vi "NML Async Lock.vi"(8 "error in (no error)":errorcluster, 11 "VISA Refnum in":refnum<visa-resource-name>) -> (0 "error out":errorcluster, 2 "Timeout":u32, 3 "VISA Refnum out":refnum<visa-resource-name>)   [LabVIEW 2025]
doc: "Gets Timeout value and Async Resource Lock. However, if connection fails it reopens connection and retrys.\nAuthor: Scott Hannahs <sth@magnet.fsu.edu>\n\nThis software is licensed for use under the “MIT License\"\nCopyright (c) 2025 Scott Hannahs, sth@sth@magnet.sthnet.net\n\nPermission is hereby granted, free of charge, to any person obtaining a copy of this software and associated documentation files (the \"Software\"), to deal in the Software without restriction, including without limitation the rights to use, copy, modify, merge, publish, distribute, sublicense, and/or sell copies of the Software, and to permit persons to whom the Software is furnished to do so, subject to the following conditions: The above copyright notice and this permission notice shall be included in all copies or substantial portions of the Software.\n\nTHE SOFTWARE IS PROVIDED \"AS IS\", WITHOUT WARRANTY OF ANY KIND, EXPRESS OR IMPLIED, INCLUDING BUT NOT LIMITED TO THE WARRANTIES OF MERCHANTABILITY, FITNESS FOR A PARTICULAR PURPOSE AND NONINFRINGEMENT. IN NO EVENT SHALL THE AUTHORS OR COPYRIGHT HOLDERS BE LIABLE FOR ANY CLAIM, DAMAGES OR OTHER LIABILITY, WHETHER IN AN ACTION OF CONTRACT, TORT OR OTHERWISE, ARISING FROM, OUT OF OR IN CONNECTION WITH THE SOFTWARE OR THE USE OR OTHER DEALINGS IN THE SOFTWARE."
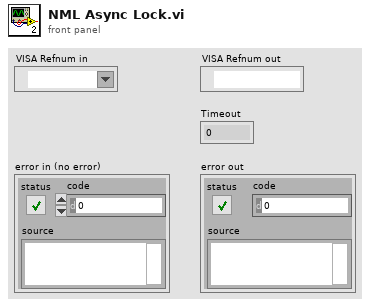
[diagram p1: front panel]
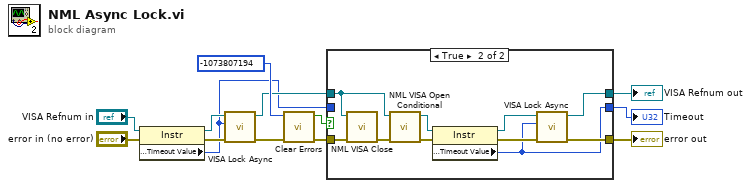
[diagram p0: block diagram]
diagram:
  n1 = property class="Instr"(reference="VISA Refnum in", error in="error in (no error)") -> (reference out=w10:refnum<visa-resource-name>, error out=w11:errorcluster, "General Settings:Timeout Value"=w1:u32)
  n2 = call <vilib>:"VISA Lock Async.vi"("error in (no error)"=w11, "timeout (0)"=w1, "VISA resource name"=w10) -> ("error out"=w8:errorcluster, "VISA resource name out"=w5:refnum<visa-resource-name>)  [unwired: 6 in, 1 out]
  n3 = call <vilib>:"Clear Errors.vi"("error in (no error)"=w8, "specific error code to clear (0: all)"=-1073807194) -> ("error out"=w6:errorcluster, "specific error cleared?"=w7:bool)  [unwired: 4 in]
  n4 = case shown="True" w7 {
    tunnel: w6 -> [w15 w26]
    tunnel: w5 -> [w16 w24]
    tunnel: [w16 w18] -> w4
    tunnel: [w15 w20] -> w3
    tunnel: [w14 w17] -> w2
    tunnel: w1 -> [w14 _]
    frame False {
    }
    frame True {
      n5 = call "NML VISA Close.vi"("Error In"=w26, "VISA resource name"=w24) -> ("Error Out"=w25:errorcluster)  [unwired: 9 in]
      n6 = call "NML VISA Open Conditional.vi"("error in (no error)"=w25, "VISA resource name"=w24) -> ("error out"=w22:errorcluster, "dup VISA Session"=w23:refnum<visa-resource-name>)  [unwired: 7 in, 1 out]
      n7 = property class="Instr"(reference=w23, error in=w22) -> (reference out=w19:refnum<visa-resource-name>, error out=w21:errorcluster, "General Settings:Timeout Value"=w17:u32)
      n8 = call <vilib>:"VISA Lock Async.vi"("error in (no error)"=w21, "timeout (0)"=w17, "VISA resource name"=w19) -> ("error out"=w20:errorcluster, "VISA resource name out"=w18:refnum<visa-resource-name>)  [unwired: 6 in, 1 out]
    }
  }
  "Timeout" <- w2
  "error out" <- w3
  "VISA Refnum out" <- w4
